vi "Form Warning Message.vi"(0 "Warnings[]":string[](array[string]), 11 "error in (no error)":errorcluster) -> (15 "error out":errorcluster)   [LabVIEW 2024, in "devicePowerSequencingModuleCoreLogic.lvlib"]
uses:
  devicePowerSequencingModuleCoreLogic.lvlib
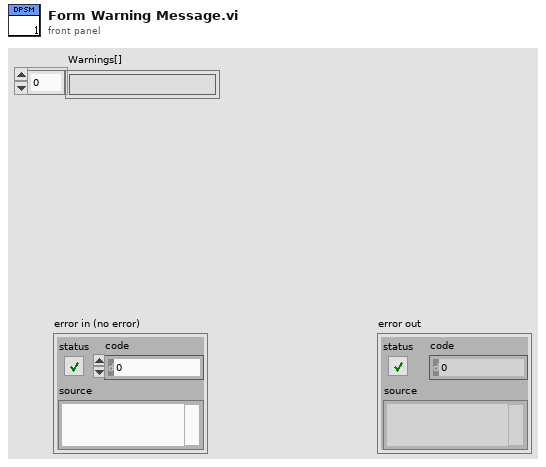
[diagram p1: front panel]
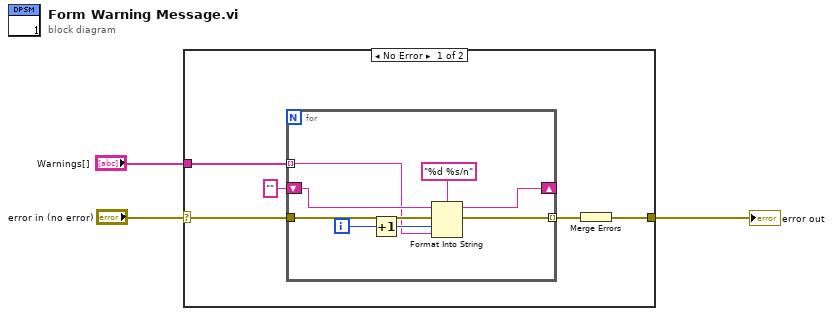
[diagram p0: block diagram]
diagram:
  n1 = case shown="No Error" "error in (no error)" {
    selector: "error in (no error)" -> [w7 w17]
    tunnel: "Warnings[]" -> [w8 _]
    tunnel: [w5 w17] -> w1
    frame No Error {
      n2 = for {
        tunnel: w8 -> [w10] mode=indexing
        tunnel: w7 -> [w16]
        tunnel: [w15] -> w6 mode=indexing
        shift-right: [w12] -> _
        shift-left: "" -> [w11]
        i -> [w14]
        n3 = Increment(x=w14) -> (x+1=w13:i32)
        n4 = Format Into String(format string="%d %s/n", initial string=w11, error in=w16, w13, w10) -> (resulting string=w12:string, error out=w15:errorcluster)
      }
      n5 = Merge Errors(w6) -> (w5:errorcluster)
    }
    frame Error {
    }
  }
  "error out" <- w1
